vi "configureTrigger_action.vi"(0 "HGF_ImaqFg":refnum<class "HGF_ImaqFg.lvclass">, 1 "Type":u32(ring) items=["External"=0, "RTSI"=1, "ISO In"=2, "Scaled Encoder"=5, "Software Trigger"=6], 2 "Line Number":u32, 3 "Frame timeout (ms)":u32=1000, 4 "Action":u32(ring) items=["Disabled", "Trigger start of acquisition", "Trigger start of each buffer list", "Trigger each buffer", "Trigger each line (linescan)", "Trigger end of acquisition"], 5 "error in (no error)":errorcluster, 6 "Activation":u32(ring) items=["Rising Edge", "Falling Edge", "AnyEdge", "LevelHigh", "LevelLow"], 7 "Delay":cluster{"Value":dbl, "Units":u32}={"Value"=0.0, "Units"=5} {"Units" items=["Scaled Encoder Counts"=4, "Milliseconds"=5]}, 8 "Mode":T1(ring), 9 "Skip trigger (linescan only)":u32) -> (14 "dup HGF_ImaqFg":refnum<class "HGF_ImaqFg.lvclass">, 19 "error out":errorcluster)   [LabVIEW 2014, in "HGF_IMAQ.lvlib" / "HGF_ImaqFg.lvclass"]
doc: "Configures the trigger conditions for an acquisition. Use this VI before any acquisition VI to setup a triggered image acquisition."
uses:
  HGF_ImaqFg.lvclass
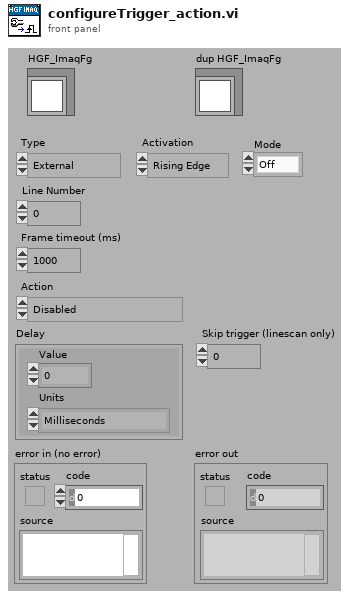
[diagram p1: front panel]
types:
  T1 = enum16{"Off", "Mode 0", "Mode 1", "Mode 2", "Mode 3", "Mode 4", "Mode 5"}
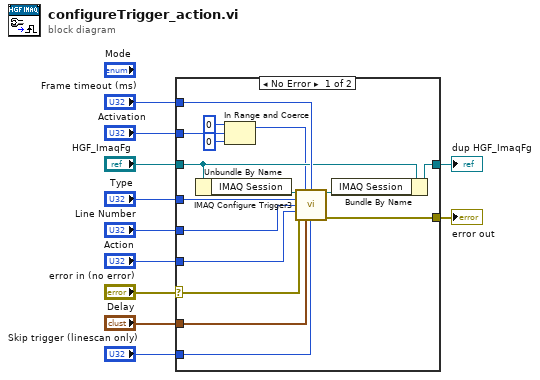
[diagram p0: block diagram]
diagram:
  n1 = case shown="No Error" "error in (no error)" {
    selector: "error in (no error)" -> [w19 w28]
    tunnel: "HGF_ImaqFg" -> [w18 w29]
    tunnel: "Activation" -> [w14 _]
    tunnel: "Frame timeout (ms)" -> [w26 _]
    tunnel: "Type" -> [w25 _]
    tunnel: "Line Number" -> [w24 _]
    tunnel: "Action" -> [w23 _]
    tunnel: "Delay" -> [w22 _]
    tunnel: "Skip trigger (linescan only)" -> [w21 _]
    tunnel: [w20 w28] -> w3
    tunnel: [w16 w29] -> w2
    frame No Error {
      n2 = Unbundle By Name(w18) -> ("IMAQ Session"=w27:refnum<k11>)
      n3 = In Range and Coerce(upper limit=u32 0, x=w14, lower limit=u32 0) -> (coerced(x)=w15:u32)  [unwired: 1 out]
      n4 = call <vilib>:"IMAQ Configure Trigger3.vi"("IMAQ Session In"=w27, "Polarity"=w15, "Frame timeout (ms)"=w26, "Type"=w25, "Line Number"=w24, "Action"=w23, "error in (no error)"=w19, "Delay"=w22, "Skip trigger (linescan only)"=w21) -> ("IMAQ Session Out"=w17:refnum<k11>, "error out"=w20:errorcluster)  [unwired: 5 in]
      n5 = Bundle By Name(cluster=w18, "IMAQ Session"=w17) -> (w16:refnum<class "HGF_ImaqFg.lvclass">)
    }
    frame Error {
    }
  }
  "error out" <- w3
  "dup HGF_ImaqFg" <- w2
